vi "VCS Get Object.vi"(0 "axis in":cluster{"keyHandle":u32, "nodeId":u16}={"keyHandle"=0, "nodeId"=1}, 5 "object in":T1 {"data" format="%x"; "object subIndex" format="%x"; "object index" format="%x"}, 11 "error in (no error)":errorcluster) -> (4 "axis out":cluster{"keyHandle":u32, "nodeId":u16}={"keyHandle"=0, "nodeId"=1}, 6 "object out":T1 {"data" format="%x"; "object subIndex" format="%x"; "object index" format="%x"}, 15 "error out":errorcluster)   [LabVIEW 2010]
doc: "<B>VCS GetObject</B> reads an object value at the given index and sub index from object dictionary."
uses:
  Resources/EposCmd.dll
  Resources/EposCmd64.dll
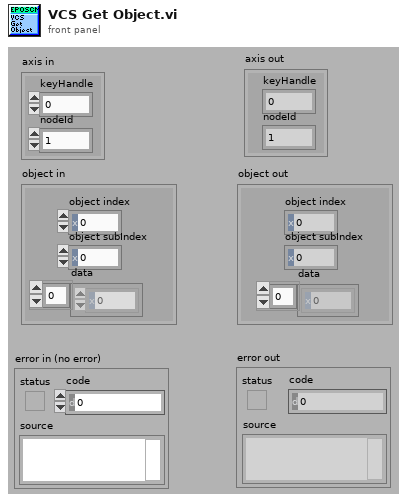
[diagram p1: front panel]
types:
  T1 = cluster{"object index":u16, "object subIndex":u8, "data":u8[]}
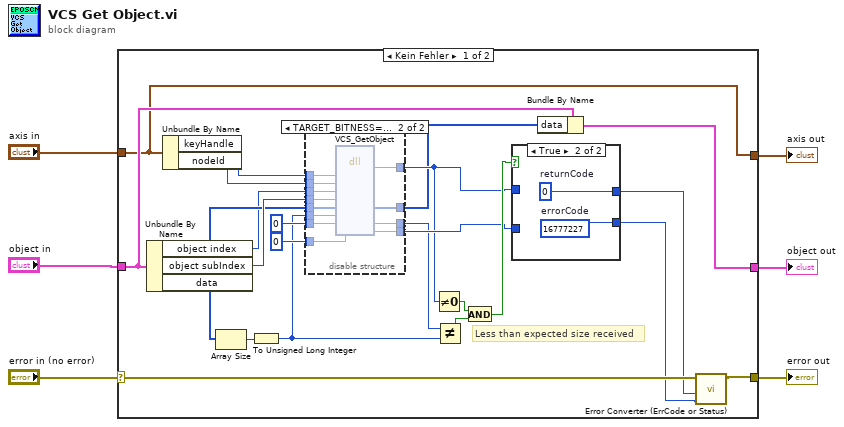
[diagram p0: block diagram]
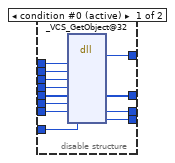
[diagram p2: hidden frame]
diagram:
  n1 = case shown="Kein Fehler" "error in (no error)" {
    selector: "error in (no error)" -> [w9 w60]
    tunnel: [w10 w60] -> w5
    tunnel: "axis in" -> [w15 w58]
    tunnel: "object in" -> [w17 w59]
    tunnel: [w19 w59] -> w3
    tunnel: [w15 w58] -> w1
    frame No Error {
      # "Less than expected size received"
      n2 = Unbundle By Name(w17) -> ("object index"=w18:u16, "object subIndex"=w27:u8, "data"=w26:u8[])
      n3 = Unbundle By Name(w15) -> ("keyHandle"=w29:u32, "nodeId"=w28:u16)
      n4 = Array Size(array=w26) -> (size(s)=w12:i32)
      n5 = To Unsigned Long Integer(number=w12) -> (unsigned 32bit integer=w11:u32)
      n6 = disable-structure shown="TARGET_BITNESS==64" {
        disable-tunnel: w29 -> [w41 w53]
        disable-tunnel: w28 -> [w40 w52]
        disable-tunnel: w27 -> [w39 w51]
        disable-tunnel: w26 -> [w38 w50]
        disable-tunnel: [w37 w49] -> w22
        disable-tunnel: [w36 w48] -> w21
        disable-tunnel: [w35 w47] -> w20
        disable-tunnel: w18 -> [w34 w46]
        disable-tunnel: [w33 w45] -> w16
        disable-tunnel: u32 0 ("pNbOfBytesRead") -> [w32 w44]
        disable-tunnel: u32 0 ("pErrorCode") -> [w31 w43]
        disable-tunnel: w11 -> [w30 w42]
        frame condition #0 (active) {
          n7 = dll-call lib="C:/Sources/LabView/maxon EPOS/Resources/EposCmd.dll" fn="_VCS_GetObject@32"("KeyHandle"=w41, "NodeId"=w40, "ObjectIndex"=w34, "ObjectSubIndex"=w39, "pData"=w38, "NbOfBytesToRead"=w30, "pNbOfBytesRead"=w32, "pErrorCode"=w31) -> ("return type"=w35:i32, "pData"=w33:u8[], "pNbOfBytesRead"=w36:u32, "pErrorCode"=w37:u32)  [unwired: 8 in, 2 out]
        }
        frame condition #1 {
          n8 = dll-call lib="C:/LabVIEW/maxon EPOS/Resources/EposCmd64.dll" fn="VCS_GetObject" ("EposCmd.dll:_VCS_GetObject@32")("KeyHandle"=w53, "NodeId"=w52, "ObjectIndex"=w46, "ObjectSubIndex"=w51, "pData"=w50, "NbOfBytesToRead"=w42, "pNbOfBytesRead"=w44, "pErrorCode"=w43) -> ("Rückgabetyp"=w47:i32, "pData"=w45:u8[], "pNbOfBytesRead"=w48:u32, "pErrorCode"=w49:u32)  [unwired: 8 in, 2 out]
        }
      }
      n9 = Not Equal To 0?(x=w20) -> (x != 0?=w24:bool)
      n10 = Not Equal?(x=w21, y=w11) -> (x != y?=w25:bool)
      n11 = And(x=w24, y=w25) -> (x .and. y?=w23:bool)
      n12 = case shown="True" w23 {
        tunnel: [w55 w57] -> w8
        tunnel: [w54 w56] -> w7
        tunnel: w20 -> [w55 _]
        tunnel: w22 -> [w54 _]
        frame False {
        }
        frame True {
          w56 = u32 16777227  # errorCode
          w57 = 0  # returnCode
        }
      }
      n13 = Bundle By Name(cluster=w17, "data"=w16) -> (w19:T1)
      n14 = call "Error Converter (ErrCode or Status).vi"("error code"=w7, "return type"=w8, "error in (no error)"=w9) -> ("error out"=w10:errorcluster)  [unwired: 7 in]
    }
    frame Error {
    }
  }
  "error out" <- w5
  "axis out" <- w1
  "object out" <- w3
